vi "Write 1Pin 1Samp Boolean.vi"(8 "error in (no error)":errorcluster, 9 "data":bool, 10 "Pin":u8, 11 "MicroDAQ.lvlib:Digital output.lvclass":refnum<class "Digital output.lvclass">) -> (0 "error out":errorcluster, 3 "MicroDAQ.lvlib:Digital output.lvclass out":refnum<class "Digital output.lvclass">)   [LabVIEW 2009, in "MicroDAQ.lvlib" / "Digital output.lvclass"]
doc: "Writes a single Boolean sample to a digital output channel composed of a single line."
uses:
  <instrlib>/MicroDAQ/Channel/Digital output/Digital output.lvclass
  <instrlib>/MicroDAQ/Channel/Channel.lvclass
  <instrlib>/MicroDAQ/Mlink library wraper/mlink.lvlib
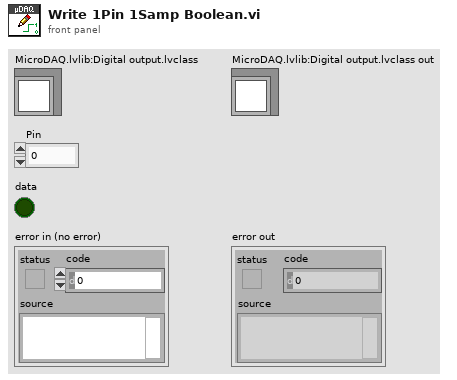
[diagram p1: front panel]
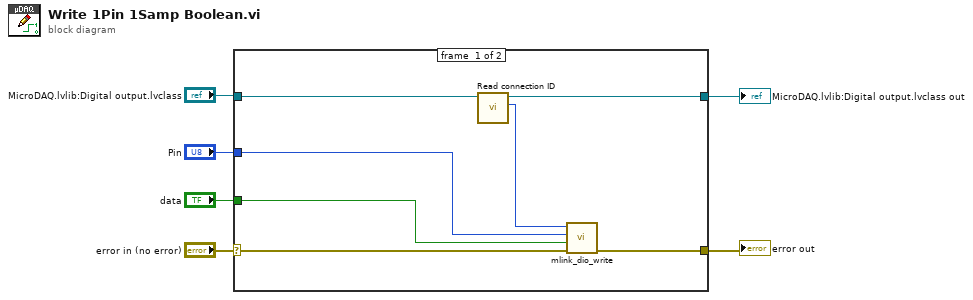
[diagram p0: block diagram]
diagram:
  n1 = case shown="No Error" "error in (no error)" {
    selector: "error in (no error)" -> [w10 w14]
    tunnel: [w11 w14] -> w5
    tunnel: "MicroDAQ.lvlib:Digital output.lvclass" -> [w12 w15]
    tunnel: [w13 w15] -> w2
    tunnel: "Pin" -> [w8 _]
    tunnel: "data" -> [w7 _]
    frame #0 {
      n2 = call <instrlib>:"Read connection ID.vi"("Task in"=w12) -> ("connection ID"=w9:i32, "Task out"=w13:refnum<class "Digital output.lvclass">)  [unwired: 9 in]
      n3 = call <instrlib>:"mlink_dio_write.vi"("error in (no error)"=w10, "state"=w7, "pin"=w8, "connection ID"=w9) -> ("error out"=w11:errorcluster)  [unwired: 6 in, 1 out]
    }
    frame #1 {
    }
  }
  "error out" <- w5
  "MicroDAQ.lvlib:Digital output.lvclass out" <- w2
